vi "PCP Voltage AND resistance value read.vi"(1 "Action(GET)":enum16{"GET", "SET"}(ring), 5 "PCP resistance":dbl, 7 "PCP voltage":dbl, 11 "error in (no error)":errorcluster) -> (6 "PCP resistance out 2":dbl, 8 "PCP voltage out":dbl, 15 "error out":errorcluster)   [LabVIEW 2011]
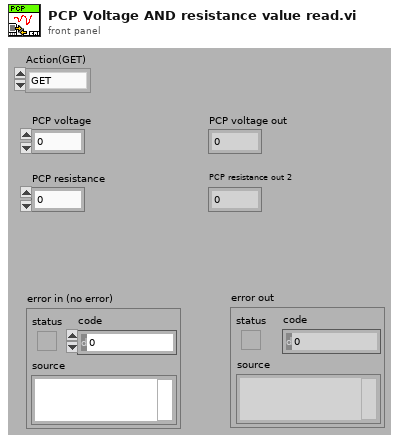
[diagram p1: front panel]
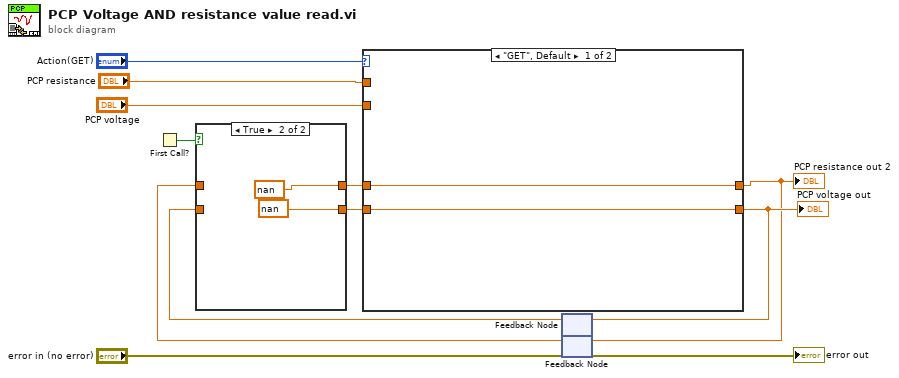
[diagram p0: block diagram]
diagram:
  n1 = First Call?() -> (First Call?: T/F=w8:bool)
  n2 = feedback #1() -> (w9:dbl)  [unwired: 1 in]
  n3 = feedback #2() -> (w1:dbl)  [unwired: 1 in]
  n4 = case shown="True" w8 {
    tunnel: w9 -> [w13 _]
    tunnel: [w13 nan ("Tool connected")] -> w6
    tunnel: [w12 nan ("Tool connected")] -> w3
    tunnel: w1 -> [w12 _]
    frame False {
    }
    frame True {
    }
  }
  n5 = case shown="\"GET\", Default" "Action(GET)" {
    tunnel: [w17 w19] -> w7
    tunnel: w6 -> [w17 _]
    tunnel: "PCP voltage" -> [_ w19]
    tunnel: "PCP resistance" -> [_ w18]
    tunnel: [w16 w18] -> w2
    tunnel: w3 -> [w16 _]
    frame "GET", Default {
    }
    frame "SET" {
    }
  }
  "PCP voltage out" <- w7
  "PCP resistance out 2" <- w2
  n6 = feedback-in #1(w7) -> ()
  n7 = feedback-in #2(w2) -> ()
  "error out" <- "error in (no error)"
